vi "setComment.vi"(8 "error in (no error)":errorcluster, 10 "comment":string, 11 "SingleToneRamp.lvclass in":refnum<class "SingleToneRamp.lvclass">) -> (0 "error out":errorcluster, 3 "SingleToneRamp.lvclass out":refnum<class "SingleToneRamp.lvclass">)   [LabVIEW 2011, in "Tools.lvlib" / "Scripting.lvlib" / "SingleToneRamp.lvclass"]
uses:
  SingleToneRamp.lvclass
  SingleTone.lvclass
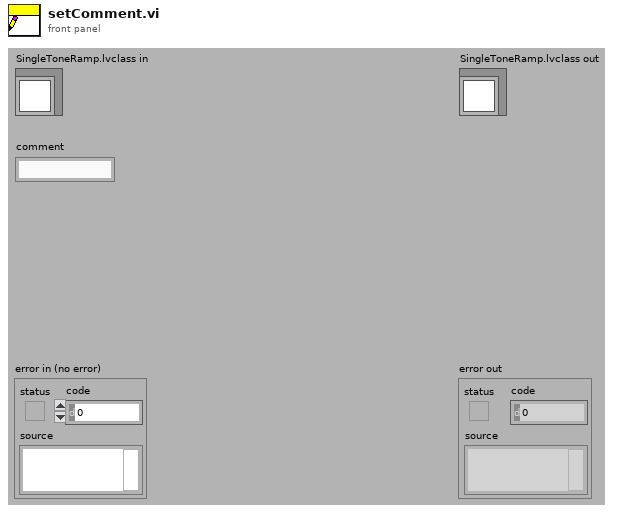
[diagram p1: front panel]
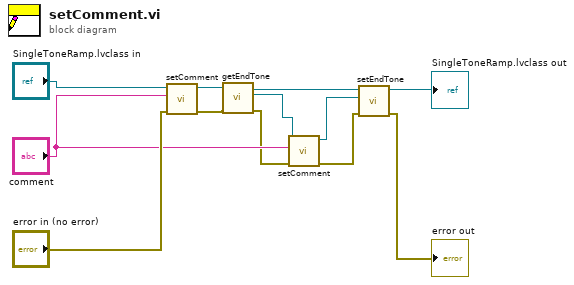
[diagram p0: block diagram]
diagram:
  n1 = call-parent "setComment.vi"("error in (no error)"="error in (no error)", "comment"="comment", "ScriptEvent.lvclass in"="SingleToneRamp.lvclass in") -> ("error out"=w10:errorcluster, "ScriptEvent.lvclass out"=w11:refnum<class "SingleToneRamp.lvclass">)  [unwired: 7 in]
  n2 = call "getEndTone.vi"("error in (no error)"=w10, "SingleToneRamp.lvclass in"=w11) -> ("error out"=w1:errorcluster, "endTone"=w3:refnum<class "SingleTone.lvclass">, "SingleToneRamp.lvclass out"=w8:refnum<class "SingleToneRamp.lvclass">)  [unwired: 7 in]
  n3 = call-dynamic "setComment.vi"("error in (no error)"=w1, "comment"="comment", "ScriptEvent.lvclass in"=w3) -> ("error out"=w5:errorcluster, "ScriptEvent.lvclass out"=w4:refnum<class "SingleTone.lvclass">)  [unwired: 7 in]
  n4 = call "setEndTone.vi"("error in (no error)"=w5, "EndTone"=w4, "SingleToneRamp.lvclass in"=w8) -> ("error out"=→"error out":errorcluster, "SingleToneRamp.lvclass out"=→"SingleToneRamp.lvclass out":refnum<class "SingleToneRamp.lvclass">)  [unwired: 7 in]
